vi "Add.vi"(8 "error in (no error)":errorcluster, 11 "subpanel (abstract) in":refnum<class "subpanel (abstract).lvclass">) -> (0 "error out":errorcluster, 3 "subpanel (abstract) out":refnum<class "subpanel (abstract).lvclass">)   [LabVIEW 2023, in "GUI.lvlib" / "subpanel (abstract).lvclass"]
uses:
  subpanel (abstract).lvclass
  subpanel (abstract).lvclass/subpanel (abstract).ctl
  plugins/modules/beamModule.vi
  GUI.lvlib
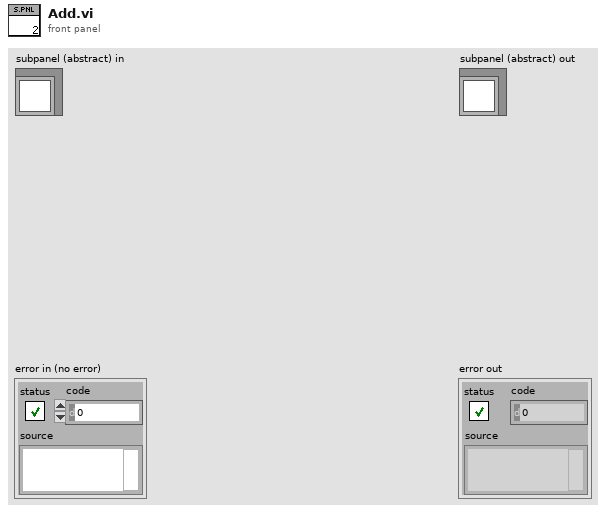
[diagram p1: front panel]
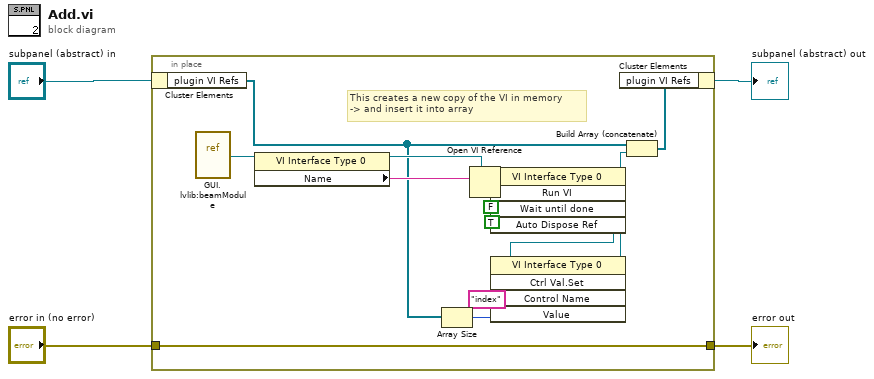
[diagram p0: block diagram]
diagram:
  n1 = in-place {
    in-place-border: "error in (no error)" -> [w17]
    in-place-border: [w17] -> w1
    # "This creates a new copy of the VI in memory \n-> and insert it into array"
    n2 = in-place-cluster #1("subpanel (abstract) in") -> ("plugin VI Refs"=w7:refnum<vi>[])
    n3 = vi-ref "GUI.lvlib:beamModule.vi"() -> (w5:refnum<vi>)
    n4 = property class="VI Interface Type 0"(reference=w5) -> (reference out=w9:refnum<vi>, "Name"=w8:string)  [unwired: 1 in, 1 out]
    n5 = Array Size(array=w7) -> (size(s)=w10:i32)
    n6 = Open VI Reference(type specifier VI Refnum (for type only)=w9, vi path=w8) -> (vi reference=w15:refnum<vi>)  [unwired: 4 in, 1 out]
    n7 = invoke class="VI Interface Type 0" method="Run VI"(reference=w15, "Wait until done"=FALSE ("Wait Until Done"), "Auto Dispose Ref"=TRUE ("Auto Dispose Reference")) -> (reference out=w12:refnum<vi>)  [unwired: 2 in, 4 out]
    n8 = invoke class="VI Interface Type 0" method="Ctrl Val.Set"(reference=w12, "Control Name"="index", "Value"=w10) -> (reference out=w11:refnum<vi>)  [unwired: 2 in, 4 out]
    n9 = Build Array (concatenate)(w7, w11) -> (w6:refnum<vi>[])
    n10 = in-place-cluster #1("plugin VI Refs"=w6) -> (→"subpanel (abstract) out":refnum<class "subpanel (abstract).lvclass">)
  }
  "error out" <- w1
